vi "DSP.vi"(0 "System no.":i32=1 min=1 max=4 step=1, 2 "DSP axes":string[](array[string]), 3 "All Axes?":bool, 4 "Axis Identifier?":bool=TRUE, 5 "error in":errorcluster) -> (19 "error out":errorcluster)   [LabVIEW 2026]
doc: "Displays selected axes on the controller screen.\n\nC-702: If All axes = TRUE, then Axis identifier must be TRUE\nC-848: If All axes = TRUE, then Axis identifier must be TRUE\nC-880: If All axes = TRUE, then Axis identifier must be TRUE"
panel:
  # "Displays selected axes on the controller screen."
  # "If all axes: use"
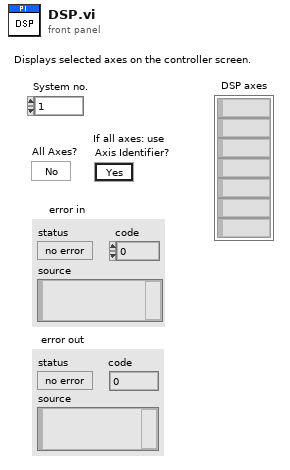
[diagram p1: front panel]
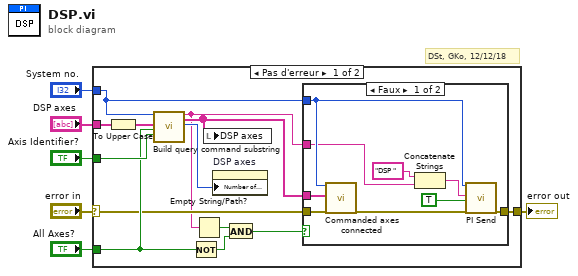
[diagram p0: block diagram]
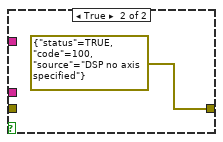
[diagram p2: hidden frame]
diagram:
  # "DSt, GKo, 12/12/18"
  n1 = case shown="Pas d'erreur" "error in" {
    selector: "error in" -> [w10 w30]
    tunnel: "DSP axes" -> [w19 _]
    tunnel: "Axis Identifier?" -> [w17 _]
    tunnel: "System no." -> [w16 _]
    tunnel: "All Axes?" -> [w13 _]
    tunnel: [w11 w30] -> w2
    frame No Error {
      n2 = To Upper Case(1:w19) -> (0:w18:string[])
      n3 = call "Build query command substring.vi"("System no."=w16, "Axes to query in"=w18, "Query\nAll axes?"=w13, "For all axes: use\nAxis identifier?"=w17) -> ("Command substring"=w9:string, "Axes to query out"=w15:string[], "Number of rows"=w14:u32)  [unwired: 2 in, 11 out]
      n4 = Not(x=w13) -> (.not. x?=w12:bool)
      n5 = Empty String/Path?(string/path=w9) -> (empty?=w8:bool)
      n6 = local write "DSP axes"(w15) -> ()
      n7 = property on="DSP axes" class="Tabl (strict)"("Number of Rows"=w14) -> ()  [unwired: 2 in, 2 out]
      n8 = And(x=w8, y=w12) -> (x .and. y?=w7:bool)
      n9 = case shown="Faux" w7 {
        tunnel: w16 -> [w25 _]
        tunnel: w15 -> [w24 _]
        tunnel: [w20 errorcluster {"status"=TRUE, "code"=100, "source"="DSP no axis specified"} ("error out")] -> w11
        tunnel: w10 -> [w22 _]
        tunnel: w9 -> [w21 _]
        frame False {
          n10 = call "Commanded axes connected.vi"("System no."=w25, "Commanded axes"=w24, "error in"=w22) -> ("error out"=w23:errorcluster)  [unwired: 1 in, 15 out]
          n11 = Concatenate Strings("DSP ", w21) -> (w26:string)
          n12 = call "PI Send.vi"("System no."=w25, "String to send"=w26, "Attach termination char.?"=TRUE ("Attach Linefeed?"), "error in"=w23) -> ("error out"=w20:errorcluster)  [unwired: 2 in, 13 out]
        }
        frame True {
        }
      }
    }
    frame Error {
    }
  }
  "error out" <- w2
